vi "LESSON3_DEBUGGING_TECHNIQUES.vi"() -> ()   [LabVIEW 2022 SP3]
panel:
  out "Numeric 3":dbl
  in  "Numeric 2":dbl
  in  "Numeric":dbl
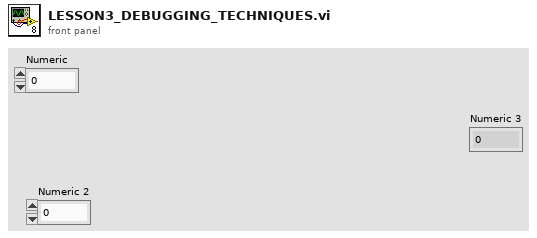
[diagram p1: front panel]
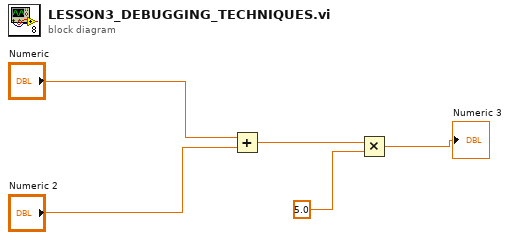
[diagram p0: block diagram]
diagram:
  n1 = Add(x="Numeric", y="Numeric 2") -> (x+y=w3:dbl)
  n2 = Multiply(x=w3, y=5.0 ("x*y")) -> (x*y=→"Numeric 3":dbl)
